vi "Move child position calc.vi"(8 "Index to move":i32, 9 "Insertion Parent Tag Index":i32, 10 "Insertion Position":i32, 11 "TreeItems":T1[](array[typedef])) -> (2 "Insertion Position (next loop)":i32)   [LabVIEW 2020, in "BetterDragAndDrop.lvlib" / "BetterTreeHandle.lvclass"]
uses:
  BetterTreeHandle/BetterTreeHandle.lvclass
  TreeItem.ctl
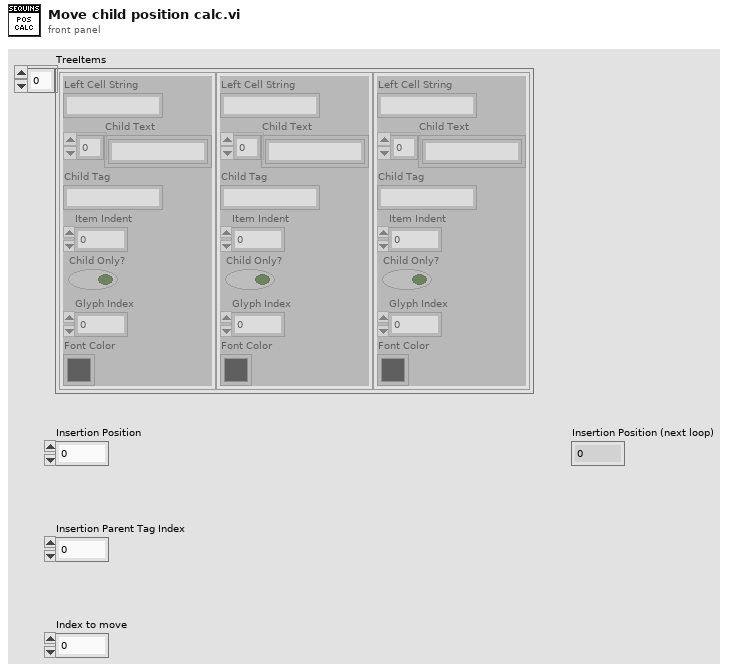
[diagram p1: front panel]
types:
  T1 = typedef "BetterDragAndDrop.lvlib/BetterTreeHandle.lvclass/TreeItem.ctl" = cluster{"Left Cell String":string, "Child Text":string[], "Child Tag":string, "Item Indent":i32, "Child Only?":bool, "Glyph Index":i32, "Font Color":u32}
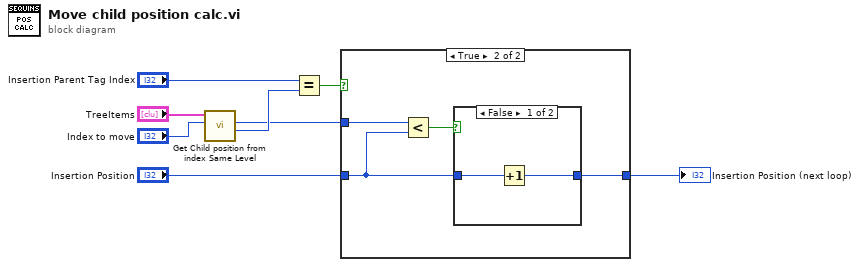
[diagram p0: block diagram]
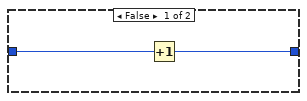
[diagram p2: hidden frame]
diagram:
  n1 = call "Get Child position from index Same Level.vi"("TreeItem Index"="Index to move", "TreeItems"="TreeItems") -> ("Parent Tag Index"=w2:i32, "Child Position"=w1:i32)  [unwired: 7 in, 1 out]
  n2 = Equal?(x="Insertion Parent Tag Index", y=w2) -> (x = y?=w7:bool)
  n3 = case shown="True" w7 {
    tunnel: "Insertion Position" -> [w10 w12]
    tunnel: [w9 w11] -> w5
    tunnel: w1 -> [_ w14]
    frame False {
      n4 = Increment(x=w10) -> (x+1=w9:i32)
    }
    frame True {
      n5 = Less?(x=w14, y=w12) -> (x < y?=w13:bool)
      n6 = case shown="False" w13 {
        tunnel: w12 -> [w16 w17]
        tunnel: [w15 w17] -> w11
        frame False {
          n7 = Increment(x=w16) -> (x+1=w15:i32)
        }
        frame True {
        }
      }
    }
  }
  "Insertion Position (next loop)" <- w5
